vi "Mixed Sample.vi"() -> (0 "Mixed Sample (Sample In: true)":refnum<class "Sample.lvclass">)   [LabVIEW 2015, in "Sample.lvclass"]
uses:
  Sample.lvclass
  Sample.lvclass/Sample.ctl
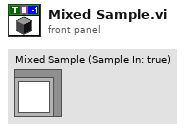
[diagram p1: front panel]
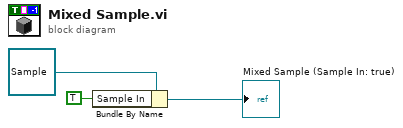
[diagram p0: block diagram]
diagram:
  n1 = Bundle By Name(cluster=refnum<class "Sample.lvclass"> refnum ("Mixed Sample (Sample In: true)"), "Sample In"=TRUE ("Sample in")) -> (→"Mixed Sample (Sample In: true)":refnum<class "Sample.lvclass">)
